vi "Refresh Token.vi"(11 "Async Authorization in":refnum<class "Async Authorization.lvclass">) -> (2 "Refresh Token":string)   [LabVIEW 2020, in "OAuth2.lvlib" / "Async Authorization.lvclass"]
uses:
  Async Authorization.lvclass
  Async Authorization.lvclass/Async Authorization.ctl
  Authorization/Authorization.lvclass
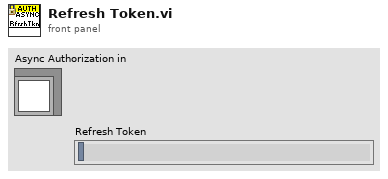
[diagram p1: front panel]
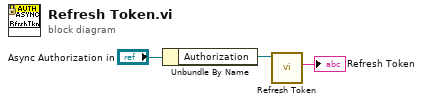
[diagram p0: block diagram]
diagram:
  n1 = Unbundle By Name("Async Authorization in") -> ("Authorization"=w2:refnum<class "Authorization.lvclass">)
  n2 = call "Refresh Token.vi"("Authorization in"=w2) -> ("Refresh Token"=→"Refresh Token":string)  [unwired: 10 in]
